vi "PathPlanner_PathFinder_DefaultNodeInfo.vi"() -> (1 "fieldWidth_Meters":i32, 2 "fieldLength_Meters":i32, 3 "NodeSize_Meters":dbl)   [LabVIEW 2019, in "PathPlanner24.lvlib"]
doc: "Internal function. Not to be used by end users."
uses:
  PathPlanner24.lvlib
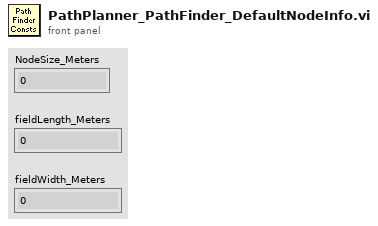
[diagram p1: front panel]
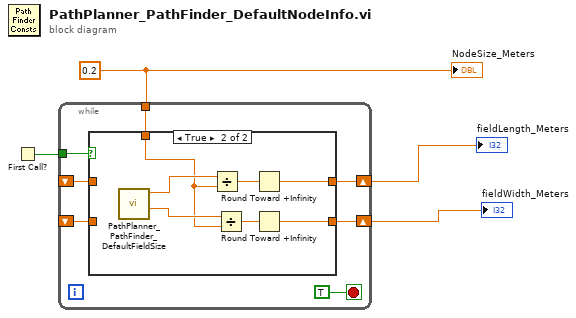
[diagram p0: block diagram]
diagram:
  w3 = 0.2 ("NodeSize_Meters")
  n1 = First Call?() -> (First Call?: T/F=w4:bool)
  n2 = while {
    tunnel: w4 -> [w10]
    tunnel: w3 -> [w9]
    shift-right: [w8] -> w2
    shift-left: _ -> [w6]
    shift-right: [w7] -> w1
    shift-left: _ -> [w5]
    stop <- TRUE stop-if-true
    n3 = case shown="True" w10 {
      tunnel: w9 -> [_ w16]
      tunnel: [w13 w15] -> w8
      tunnel: [w12 w14] -> w7
      tunnel: w6 -> [w13 _]
      tunnel: w5 -> [w12 _]
      frame False {
      }
      frame True {
        n4 = call "PathPlanner_PathFinder_DefaultFieldSize.vi"() -> ("fieldWidth_Meters"=w19:dbl, "fieldLength_Meters"=w20:dbl)  [unwired: 10 in]
        n5 = Divide(x=w20, y=w16) -> (x/y=w18:dbl)
        n6 = Divide(x=w19, y=w16) -> (x/y=w17:dbl)
        n7 = Round Toward +Infinity(x=w18) -> (ceil(x): smallest int >= x=w15:dbl)
        n8 = Round Toward +Infinity(x=w17) -> (ceil(x): smallest int >= x=w14:dbl)
      }
    }
  }
  "fieldLength_Meters" <- w2
  "fieldWidth_Meters" <- w1
  "NodeSize_Meters" <- w3
